vi "List Packages in NIPB Solution.vi"(8 "error in (no error)":errorcluster, 11 "NI Package Builder solution (.pbs)":path) -> (0 "error out":errorcluster, 2 "package names":string[](array[string]), 3 "NI Package Builder solution out":path)   [LabVIEW 2017, in "NIPB Solution API.lvlib"]
doc: "Gets the category of the specified package in the specified NI Package Builder solution (.pbs).\n\nIf the <b>package name</b> input is unwired, this VI will perform this operation on the first package in the NI Package Builder solution and output the corresponding package name in the <b>package name out</b> output."
uses:
  NIPB Solution API.lvlib
  <vilib>/xml/NI_XML.lvlib
  <vilib>/xml/Load XML File.vi
  <vilib>/xml/Close Reference(Node).vi
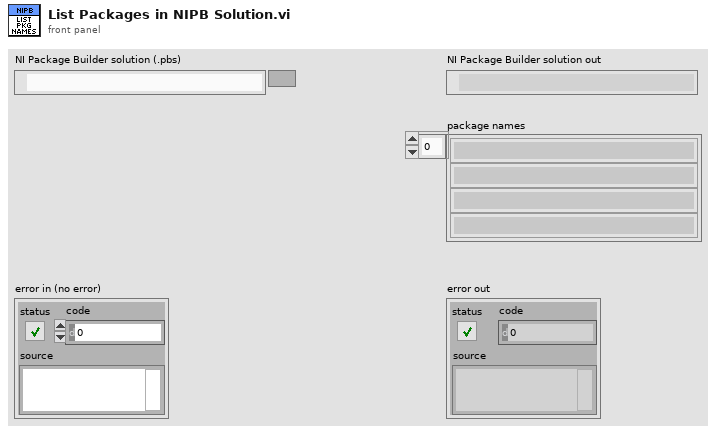
[diagram p1: front panel]
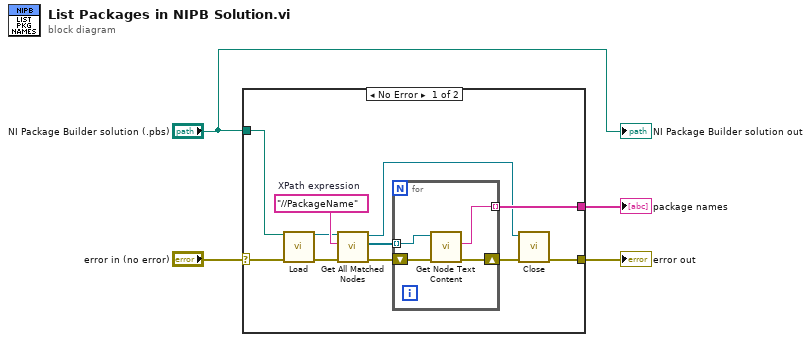
[diagram p0: block diagram]
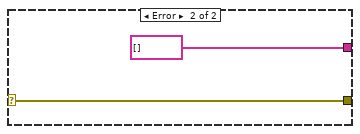
[diagram p2: hidden frame]
diagram:
  n1 = case shown="No Error" "error in (no error)" {
    selector: "error in (no error)" -> [w13 w21]
    tunnel: [w8 w21] -> w3
    tunnel: "NI Package Builder solution (.pbs)" -> [w9 _]
    tunnel: [w7 string[] []] -> w1
    frame No Error {
      w15 = "//PackageName"  # XPath expression
      n2 = call-poly <vilib>:"Load.vi"("path to XML document"=w9, "error in (no error)"=w13) -> ("DOM document out"=w10:refnum<k20>, "error out"=w14:errorcluster)  [unwired: 11 in, 1 out]
      n3 = call <vilib>:"Get All Matched Nodes.vi"("error in (no error)"=w14, "XPath expression"=w15, "node in"=w10) -> ("error out"=w12:errorcluster, "node result array"=w6:refnum<k20>[], "node out"=w5:refnum<k20>)  [unwired: 6 in]
      n4 = for {
        shift-right: [w18] -> w11
        shift-left: w12 -> [w19]
        tunnel: [w17] -> w7 mode=indexing
        tunnel: w6 -> [w16] mode=indexing
        n5 = call <vilib>:"Get Node Text Content.vi"("error in (no error)"=w19, "node in"=w16) -> ("error out"=w18:errorcluster, "node text"=w17:string)  [unwired: 7 in, 1 out]
      }
      n6 = call-poly <vilib>:"Close.vi"("error in (no error)"=w11, "node"=w5) -> ("error out"=w8:errorcluster)  [unwired: 7 in]
    }
    frame Error {
    }
  }
  "error out" <- w3
  "package names" <- w1
  "NI Package Builder solution out" <- "NI Package Builder solution (.pbs)"
